vi "Read Measurements.vi"(8 "error in (no error)":errorcluster, 11 "NhRegenGridSim in":refnum<class "NHRGridSim.lvclass">) -> (0 "error out":errorcluster, 2 "Measurements":T1 {"Phase" items=["All", "A Phase", "B Phase", "C Phase"]}, 3 "NhRegenGridSim out":refnum<class "NHRGridSim.lvclass">)   [LabVIEW 2018, in "AcPwrPlugins.lvlib" / "NHRGridSim.lvclass"]
uses:
  NHRGridSim.lvclass
  PublicMethods/Measurements.ctl
  TypeDefs/MeasurementType.ctl
  NHRGridSim.lvclass/NHRGridSim.ctl
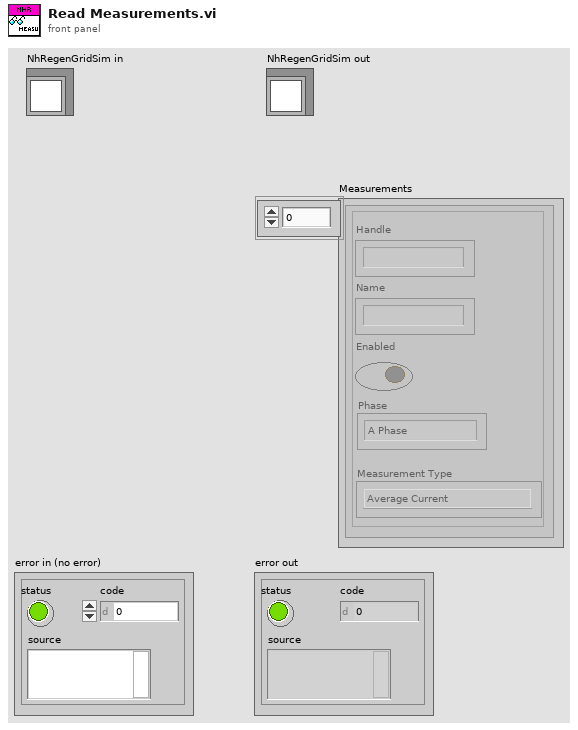
[diagram p1: front panel]
types:
  T1 = typedef "AcPwrPlugins.lvlib/NHRGridSim.lvclass/Measurements.ctl" = cluster{"Handle":string, "Name":string, "Enabled ":bool, "Measurement Value":dbl, "Phase ":i32, "Measurement Type ":T2}[]
  T2 = typedef "AcPwrPlugins.lvlib/NHRGridSim.lvclass/MeasurementType.ctl" = enum16{"Average Current", "Average Voltage"}
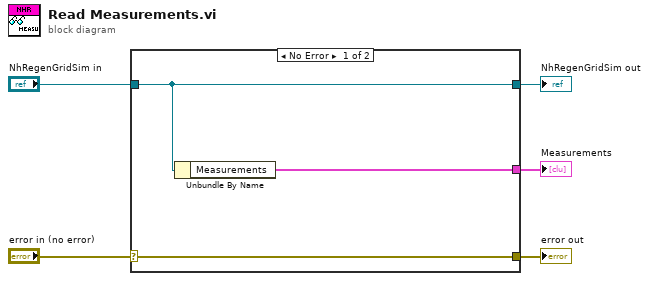
[diagram p0: block diagram]
diagram:
  n1 = case shown="No Error" "error in (no error)" {
    selector: "error in (no error)" -> [w8 w9]
    tunnel: [w8 w9] -> w4
    tunnel: [w7 w10] -> w2
    tunnel: "NhRegenGridSim in" -> [w7 w10]
    tunnel: [w6 _] -> w1
    frame No Error {
      n2 = Unbundle By Name(w7) -> ("Measurements"=w6:T1)
    }
    frame Error {
    }
  }
  "error out" <- w4
  "NhRegenGridSim out" <- w2
  "Measurements" <- w1
